vi "Poligono.vi"() -> ()   [LabVIEW 2016]
panel:
  out "Waveform Graph 2":dbl[](graph)
  out "Waveform Graph":dbl[](graph)
  out "XY Graph":cluster{dbl[], dbl[]}(graph)
  in  "L":dbl
  # "Grados=2PI/L"
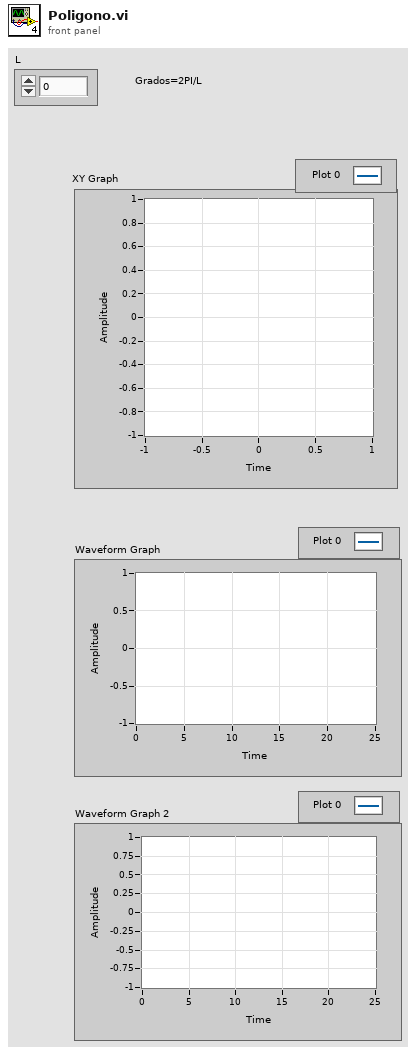
[diagram p1: front panel]
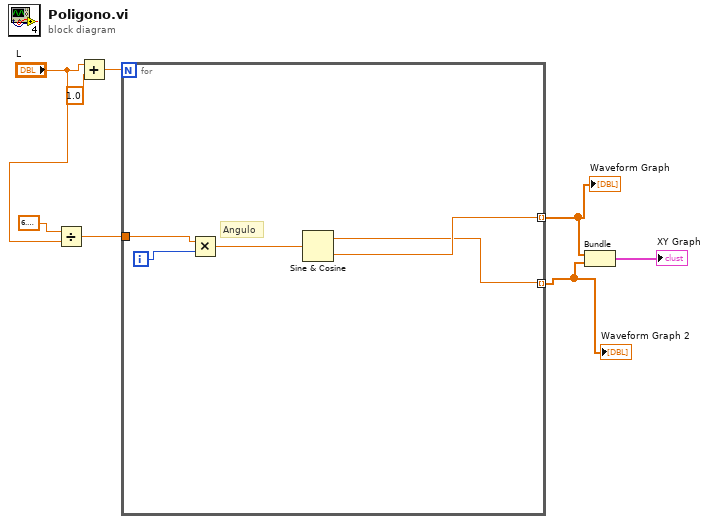
[diagram p0: block diagram]
diagram:
  n1 = Divide(x=6.283185307179586, y="L") -> (x/y=w7:dbl)
  n2 = Add(x="L", y=1.0) -> (x+y=w4:dbl)
  n3 = for {
    N: w4 -> [_]
    tunnel: w7 -> [w12]
    tunnel: [w10] -> w1 mode=indexing
    tunnel: [w9] -> w2 mode=indexing
    i -> [w13]
    # "Angulo"
    n4 = Multiply(x=w12, y=w13) -> (x*y=w11:dbl)
    n5 = Sine & Cosine(0:w11) -> (1:w9:dbl, 2:w10:dbl)
  }
  "Waveform Graph 2" <- w2
  "Waveform Graph" <- w1
  n6 = Bundle(w1, w2) -> (→"XY Graph":cluster{dbl[], dbl[]})  [unwired: 1 in]
